vi "CS++UtilitiesContent.vi"() -> (0 "CS++Classes & Messages":T1(array[cluster]))   [LabVIEW 2016]
doc: "Place actor and class constants that should be included included in an application on the blockdiagramm."
uses:
  <vilib>/ActorFramework/Message/Message.lvclass
  Actors/CS++BeepActor/Beep/Beep.lvclass
  C:/User/Brand/LVP/TASCA/UTCS/Packages/CSPP_Core/Actors/CS++BaseActor/CS++BaseActor.lvclass
  CSPP_Core/Actors/CS++BaseActor/CS++BaseActor.lvclass
panel:
  # "Place actor and class constants on the blockdiagramm."
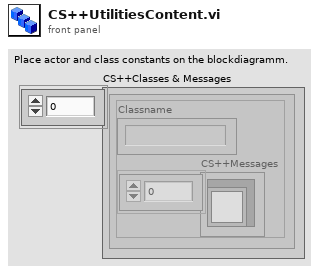
[diagram p1: front panel]
types:
  T1 = cluster{"Classname":string, "CS++Messages":refnum<class "Message.lvclass">[]}[]
  T2 = cluster{"class name":string, "CS++Messages":refnum<class "Message.lvclass">[]}
  T3 = cluster{"class name":string, "CS++Messages":refnum<class "Message.lvclass">[]}[]
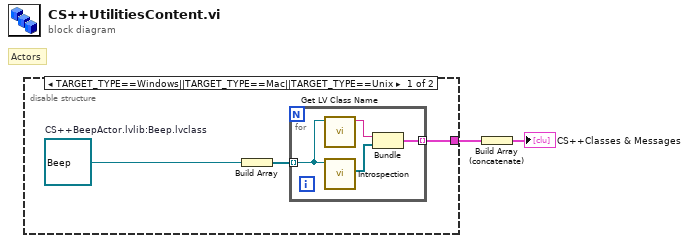
[diagram p0: block diagram]
diagram:
  # "Actors"
  n1 = disable-structure shown="TARGET_TYPE==Windows||TARGET_TYPE==Mac||TARGET_TYPE==Unix" {
    disable-tunnel: [w4 _] -> w1
    frame condition #0 (active) {
      w3 = refnum<class "Beep.lvclass"> refnum  # CS++BeepActor.lvlib:Beep.lvclass
      n2 = Build Array(w3) -> (w5:refnum<class "Beep.lvclass">[])
      n3 = for {
        tunnel: w5 -> [w9] mode=indexing
        tunnel: [w6] -> w4 mode=indexing
        n4 = call <vilib>:"Get LV Class Name.vi"("object"=w9) -> ("class name"=w8:string)  [unwired: 9 in, 1 out]
        n5 = call "Introspection.vi"("CS++BaseActor in"=w9) -> ("CS++Messages"=w7:refnum<class "Message.lvclass">[])  [unwired: 8 in, 2 out]
        n6 = Bundle("class name"=w8, "CS++Messages"=w7) -> (w6:T2)  [unwired: 1 in]
      }
    }
    frame condition #1 {
    }
  }
  n7 = Build Array (concatenate)(w1) -> (→"CS++Classes & Messages":T3)
